vi "Visa Close.vi"(8 "错误输入（无错误）":errorcluster, 10 "Mask":T1=16 items=["清空接收缓冲区"=16, "向设备写入传输缓冲区"=32, "清空接收缓冲区（无I/O）"=64, "清空传输缓冲区"=128], 11 "VISA":T2={"VISA"="", "baud rate"=9600, "data bits"=8, "parity"=enum."None", "stop bits"=10, "flow control"=0} {"flow control" items=["无", "XON/XOFF", "RTS/CTS", "XON/XOFF & RTS/CTS", "DTR/DSR", "XON/XOFF & DTR/DSR"]; "stop bits" items=["1.0"=10, "1.5"=15, "2.0"=20]; "data bits" min=5 max=8 step=1}) -> (0 "错误输出":errorcluster)   [LabVIEW 2014]
uses:
  <vilib>/Instr/_visa.llb/VISA Flush IO Buffer Mask.ctl
  Ctr/VISA Ctr.ctl
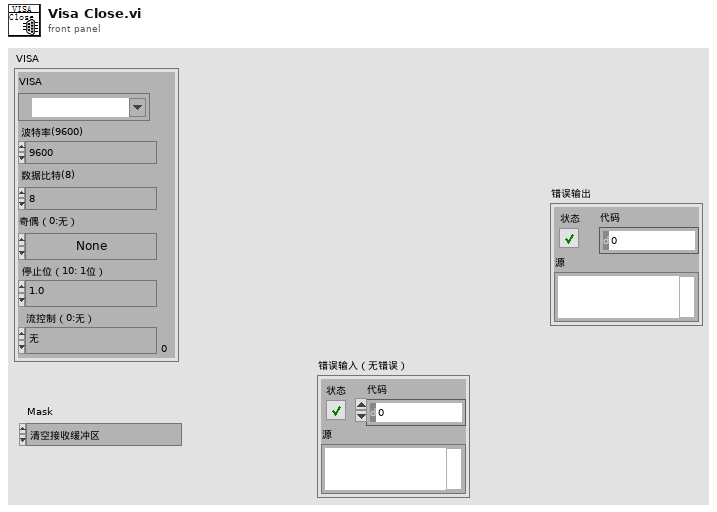
[diagram p1: front panel]
types:
  T1 = typedef "VISA Flush IO Buffer Mask.ctl" = u16
  T2 = typedef "VISA Ctr.ctl" = cluster{"VISA":refnum<visa-resource-name>, "baud rate":u32, "data bits":u16, "parity":enum16{"None", "Odd", "Even", "Mark", "Space"}, "stop bits":u16, "flow control":u16}
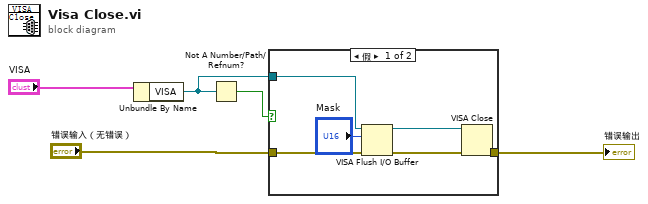
[diagram p0: block diagram]
diagram:
  n1 = Unbundle By Name("VISA") -> ("VISA"=w1:refnum<visa-resource-name>)
  n2 = Not A Number/Path/Refnum?(number/path/refnum=w1) -> (NaN/Path/Refnum?=w2:bool)
  n3 = case shown="假" w2 {
    tunnel: "错误输入（无错误）" -> [w9 w12]
    tunnel: [w8 w12] -> w4
    tunnel: w1 -> [w6 _]
    frame False {
      n4 = VISA Flush I/O Buffer(VISA resource name=w6, mask (16)="Mask", error in (no error)=w9) -> (VISA resource name out=w10:refnum<visa-resource-name>, error out=w11:errorcluster)
      n5 = VISA Close(VISA resource name=w10, error in (no error)=w11) -> (error out=w8:errorcluster)
    }
    frame True {
    }
  }
  "错误输出" <- w4
